vi "Start Proxy.vi"(0 "Sift Client in":refnum<class "Sift Client.lvclass">, 1 "Num. Ingestion Workers":u8=1, 5 "Storage Path":path, 11 "error in (no error)":errorcluster) -> (4 "Sift Client out":refnum<class "Sift Client.lvclass">, 15 "error out":errorcluster)   [LabVIEW 2024, in "Sift Client.lvlib" / "Sift Client.lvclass"]
doc: "Starts Sift Proxy. This should only be called if Sift Proxy is not already running.\n\nLogs and data that failed to upload will be saved in Storage Path.\n\nNum Ingestion Workers can be set to increase the throughput of data sent to Sift."
uses:
  Sift Client.lvclass
  Sift Client.lvclass/Sift Client.ctl
  <vilib>/Utility/error.llb/Error Cluster From Error Code.vi
  <vilib>/ErrorRing/Error Ring.xnode
  <userlib>/_OpenG.lib/error/error.llb/openg_error.lvlib
panel:
  out "Executable Path":path
  out "Ping Attempts":i32
  out "Command Line":string
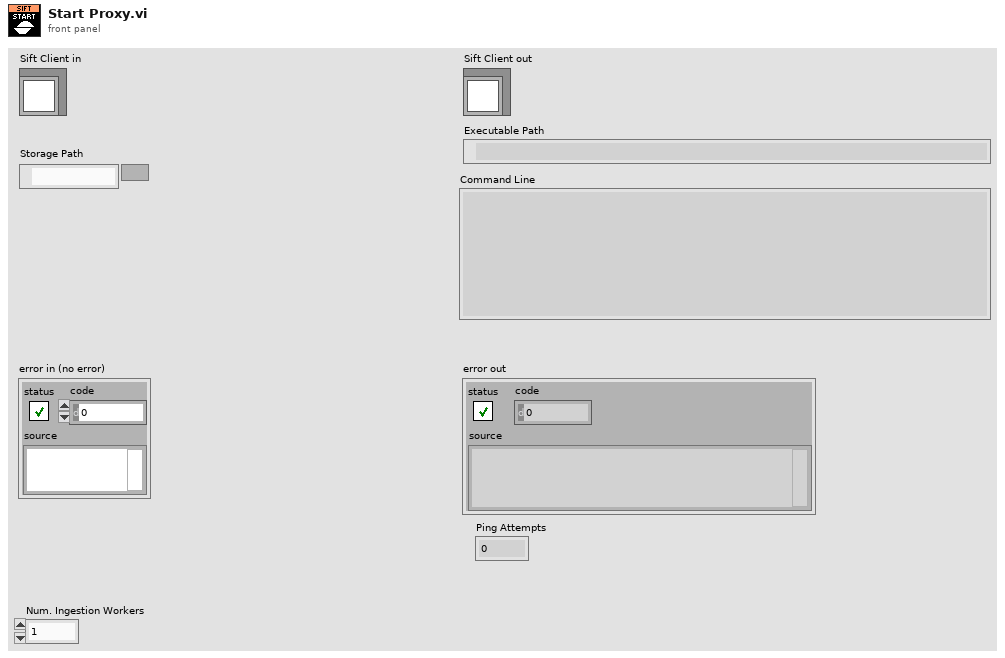
[diagram p1: front panel]
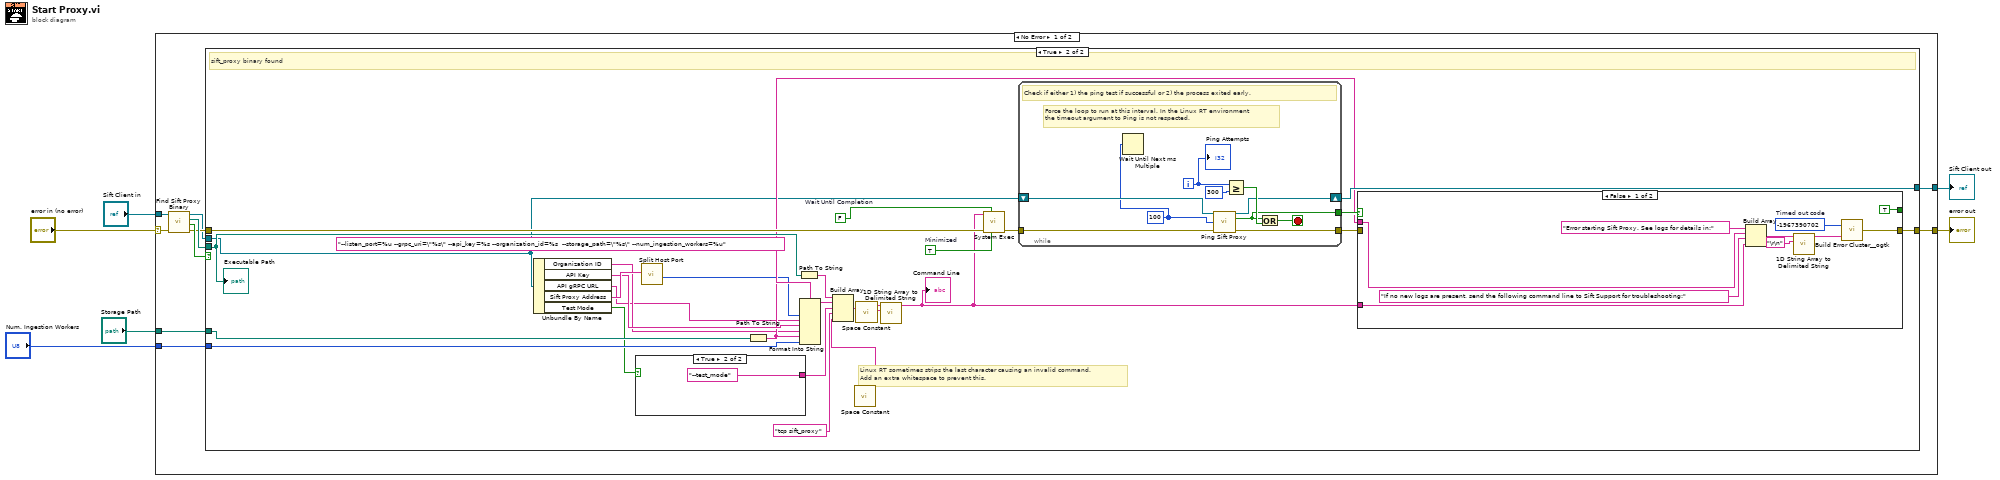
[diagram p0: block diagram]
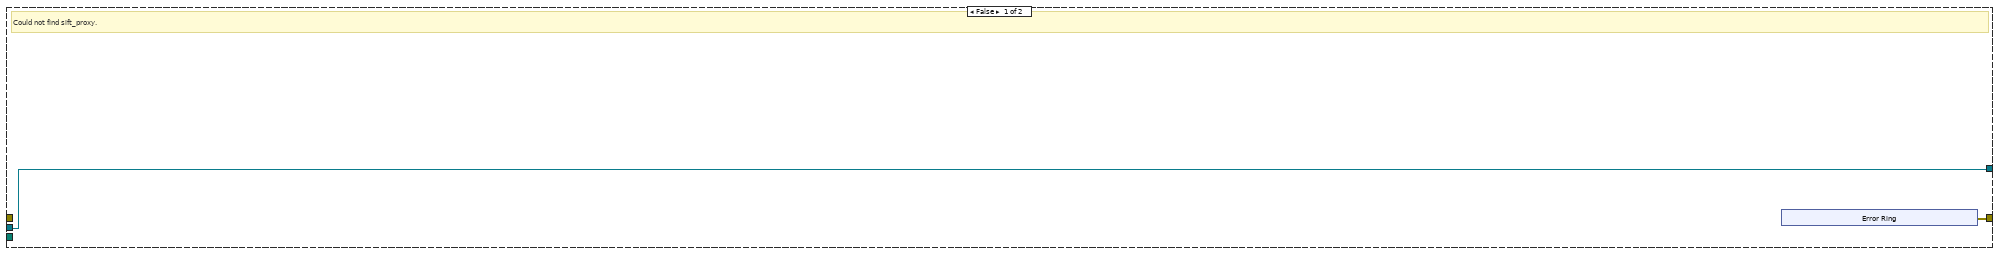
[diagram p2: hidden frame]
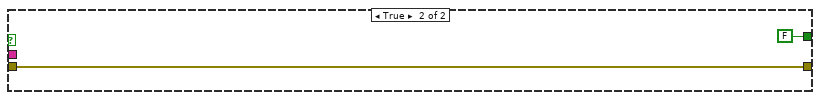
[diagram p3: hidden frame]
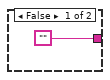
[diagram p4: hidden frame]
diagram:
  n1 = case shown="No Error" "error in (no error)" {
    selector: "error in (no error)" -> [w9 w77]
    tunnel: [w14 w76] -> w4
    tunnel: "Sift Client in" -> [w10 w76]
    tunnel: "Storage Path" -> [w16 _]
    tunnel: "Num. Ingestion Workers" -> [w15 _]
    tunnel: [w13 w77] -> w1
    frame No Error {
      n2 = call-dynamic "Find Sift Proxy Binary.vi"("error in (no error)"=w9, "Sift Client in"=w10) -> ("error out"=w8:errorcluster, "Found"=w12:bool, "Path"=w11:path, "Sift Client out"=w7:refnum<class "Sift Client.lvclass">)  [unwired: 6 in]
      n3 = case shown="True" w12 {
        tunnel: w16 -> [_ w51]
        tunnel: w15 -> [_ w35]
        tunnel: [w18 w43] -> w14
        tunnel: [w17 w50] -> w13
        tunnel: w7 -> [w18 w27]
        tunnel: w8 -> [_ w49]
        tunnel: w11 -> [_ w48]
        frame False {
          # "Could not find sift_proxy."
          n4 = xnode "Error Ring"() -> ("error out"=w17:errorcluster)
        }
        frame True {
          w42 = TRUE  # Minimized
          w46 = FALSE  # Wait Until Completion
          # "Linux RT sometimes strips the last character causing an invalid command. \nAdd an extra whitespace to prevent this."
          # "sift_proxy binary found"
          n5 = Unbundle By Name(w27) -> ("Organization ID"=w36:string, "API Key"=w38:string, "API gRPC URL"=w24:string, "Sift Proxy Address"=w40:string, "Test Mode"=w26:bool)
          n6 = case shown="True" w26 {
            tunnel: ["" "--test_mode"] -> w29
            frame False {
            }
            frame True {
            }
          }
          n7 = call "Split Host Port.vi"("Address"=w40) -> ("Port"=w39:i32)  [unwired: 9 in, 1 out]
          n8 = Path To String(path=w51) -> (string=w37:string)
          n9 = Path To String(path=w48) -> (string=w32:string)
          n10 = Format Into String(format string="--listen_port=%u --grpc_uri=\"%s\" --api_key=%s --organization_id=%s  --storage_path=\"%s\" --num_ingestion_workers=%u", w39, w24, w38, w36, w37, w35) -> (resulting string=w33:string)  [unwired: 2 in, 1 out]
          n11 = call <vilib>:"Space Constant.vi"() -> ("String"=w25:string)
          n12 = Build Array(w32, w33, w29, "tcp sift_proxy", w25) -> (w31:string[])
          n13 = call <vilib>:"Space Constant.vi"() -> ("String"=w34:string)
          n14 = call <vilib>:"1D String Array to Delimited String.vi"("delimiter"=w34, "string array"=w31) -> ("delimited string"=w28:string)  [unwired: 9 in]
          "Command Line" <- w28
          n15 = call <vilib>:"System Exec.vi"("run minimized? (F)"=w42, "wait until completion? (T)"=w46, "error in (no error)"=w49, "command line"=w28) -> ("error out"=w45:errorcluster)  [unwired: 4 in, 3 out]
          n16 = while {
            tunnel: w45 -> [w71]
            tunnel: [w70] -> w47
            tunnel: [w68] -> w44
            shift-right: [w67] -> w43
            shift-left: w27 -> [w69]
            i -> [w72]
            stop <- w74 stop-if-true
            w66 = 100
            # "Force the loop to run at this interval. In the Linux RT environment\nthe timeout argument to Ping is not respected."
            # "Check if either 1) the ping test if successful or 2) the process exited early."
            n17 = Wait Until Next ms Multiple(millisecond multiple=w66) -> ()  [unwired: 1 out]
            n18 = call-dynamic "Ping Sift Proxy.vi"("Sift Client in"=w69, "Timeout"=w66, "error in (no error)"=w71) -> ("Sift Client out"=w67:refnum<class "Sift Client.lvclass">, "Success"=w68:bool, "error out"=w70:errorcluster)  [unwired: 10 in]
            n19 = Greater Or Equal?(x=w72, y=300) -> (x >= y?=w73:bool)
            n20 = Or(x=w68, y=w73) -> (x .or. y?=w74:bool)
            "Ping Attempts" <- w72
          }
          n21 = case shown="False" w44 {
            tunnel: [w59 w63] -> w50
            tunnel: w47 -> [_ w63]
            tunnel: [TRUE FALSE] -> _
            tunnel: w37 -> [w57 _]
            tunnel: w28 -> [w55 _]
            frame False {
              w60 = -1967390702  # Timed out code
              n22 = Build Array("Error starting Sift Proxy. See logs for details in:", w57, "If no new logs are present, send the following command line to Sift Support for troubleshooting:", w55) -> (w53:string[])
              n23 = call <vilib>:"1D String Array to Delimited String.vi"("delimiter"="\r\n", "string array"=w53) -> ("delimited string"=w52:string)  [unwired: 9 in]
              n24 = call <userlib>:"Build Error Cluster__ogtk.vi"("String to Prepend to source (\"\")"=w52, "code"=w60) -> ("error out"=w59:errorcluster)
            }
            frame True {
            }
          }
          "Executable Path" <- w48
        }
      }
    }
    frame Error {
    }
  }
  "error out" <- w1
  "Sift Client out" <- w4
